vi "Modem Status data gathering Loop.vi"(1 "Loop ID":T1=enum."Var Handling-From PCP", 11 "error in":errorcluster) -> ()   [LabVIEW 2011]
uses:
  Application Structure/Loop ID.ctl
  Tool/Variable List Tool Analog.ctl
  Tool/Variable List Tool Digital.ctl
  Common/Variable List Common Digital.ctl
  Common/Variable List Common Analog.ctl
  Action Analog Handler.ctl
  Modem Status/Variable List Modem Status Digital.ctl
  Modem Status/Variable List Modem Status Analog.ctl
  Status Digitalish.ctl
  emi Lib/System 01/0 - General/App/Loop control 2/Private/_emi_ SMLoop start condition.vi
  emi Lib/System 01/0 - General/App/Loop control 2/Private/_emi_ SMLoop Error Check.vi
  emi Lib/Basic/0 - General/Error/emi_Is Error.vi
  emi Lib/System 01/0 - General/App/Loop control 2/Private/_emi_SMLoop Register new.vi
  emi Lib/System 01/0 - General/S&E reporting/emi_Send S&E Error message.vi
  emi Lib/Basic/0 - General/Error/emi_ Is Error state.vi
  emi Lib/System 01/0 - General/emi_Read System ID.vi
  emi Lib/System 01/0 - General/App/Loop control/Private/_emi_GFV Loop Linking.vi
  emi Lib/System 01/0 - General/App/Loop control/Private/_emi_GFV Loop Enable.vi
  emi Lib/System 01/0 - General/App/Loop control 2/Private/_emi_ SMLoop Restart.vi
  emi Lib/System 01/0 - General/App/Private/_emi_GFV App Close.vi
  emi Lib/System 01/0 - General/App/Loop control 2/Private/_emi_ SMLoop Restart Counter.vi
  emi Lib/System 01/0 - General/App/Loop control/Private/_emi_GFV Loop Running.vi
  emi Lib/System 01/0 - General/Private/_emi_GFV System ID.vi
  emi Lib/System 01/0 - General/S&E reporting/Private/_emi_S&E Q Generator.vi
  <vilib>/Utility/error.llb/Clear Errors.vi
  emi Lib/System 01/0 - General/App/Loop control/Private/_emi_GFV stop a loop so it can reset.vi
  <vilib>/Utility/VariantDataType/GetNumericInfo.vi
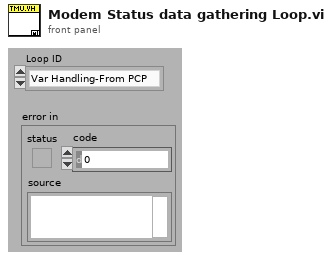
[diagram p1: front panel]
types:
  T1 = typedef "Loop ID.ctl" = enum16{"Main-QSM", "Main-Dialog", "Main-Ind Upd", "Main-Graph Upd", "Main-Debug", "Main-DebugW1", "Main-DebugW2", "Main-SE Handler", "Interface-PCP", "Interface-CANbus", "Interface-Modem", "Var Handling-Beat", "Var Handling-From PCP", "Var Handling-File storage", "Var Handling-From Simulator", "GUI-GrphW Mast", "GUI-GrphW Slav", "SIM-Tool W1", "SIM-Tool W2", "Alm-Sound", "LEIN-motor", "Tool data gatherer Qer", "Tool Data LEIN STAT2 dekoder", "Indicator Value Update", "Tool STAT2 dedicated reader", "Tool ID handler", "Detail View L1", "Detail View L2", "Main display enable view", "Sequence runner", "Voltage setpoint", "Resistance setpoint", "Stroker Wizard L1", "Stroker Wizard L2", "Alarm Handling", "Annotations Tip Strip", "Magna Interface", "Modem Status", "Var Handling - Modem Status", "Power interface detector"}
  T2 = typedef "Variable List Tool Analog.ctl" = enum16{"Tool Max Temperature", "Tool (Controller) Temperature", "Tool Supply Voltage", "Tool (Controller) Current", "Tool Acceleration X", "Tool Acceleration Y", "Tool Acceleration Z", "Tool Acceleration Sum", "Tool Inclination", "Tool Rotation", "Tool GP Sensor 1", "Tool GP Sensor 2", "Tool (Pressure 1) Temperature", "Tool Pressure 1 RAW", "Tool (Pressure 2) Temperature", "Tool Pressure 2 RAW", "Tool (Solenoid) Temperature", "Tool Solenoid Position", "PSU Temp", "Head Voltage", "PSU Main Voltage out", "PSU Main Current out", "Upper Tension Sub Temp", "Tool Upper Tension Sub Raw", "Lower Tension Sub Temp", "Tool Lower Tension Sub Raw", "Tool Var27 - Reserved", "Tool Var28 - Reserved", "Tool Var29 - Reserved", "Tool Var30 - Reserved", "Stroke Extension", "Stroke In Force", "Stroke Out Force", "Stroke Force", "Stroker Pressure 1", "Stroker Pressure 2", "Stroker Upper Tension Sub", "Stroker Lower Tension Sub", "Stroker Var09 - Reserved", "Stroker Var10 - Reserved", "Tractor Upper Tension Sub", "Tractor Lower Tension Sub", "Tractor Var03 - Reserved", "Tractor Var04 - Reserved", "Tool Temperature sensor", "Tool Motor Voltage", "Tool Motor Current", "Tool Motor Torque", "Tool weight on bit", "Tool Motor RPM"}
  T3 = typedef "Variable List Tool Digital.ctl" = enum16{"Tool Error Controller", "Tool Stopped Controller", "Tool Relay 1", "Tool Relay 2", "Tool Both Relays", "Tool node Pressure 1", "Tool Error Pressure 1", "Tool Stopped Pressure 1", "Tool node Pressure 2", "Tool Error Pressure 2", "Tool Stopped Pressure 2", "Tool node Solenoid", "Tool Error Solenoid", "Tool Stopped Solenoid", "Tool Solenoid 1", "Tool Solenoid 2", "Tool Solenoid 3", "Tool node PSU", "Tool Error PSU", "Tool Stopped PSU", "Upper Tension Sub", "Tool Error Upper Tension Sub", "Tool Stopped Upper Tension Sub", "Lower Tension Sub", "Tool Error Lower Tension Sub", "Tool Stopped Lower Tension Sub", "Stroke Target seeking", "Stroke Moving Out", "Stroke Moving Inn", "Stroke valves set for Out", "Stroke valves set for In", "Stroke In (force)", "Stroke Out (force)", "Stroke Force decreasing(in)", "Stroke Force decreasing(out)", "Stroke Force change not correct", "Stroke SLIPS established P1", "Stroke SLIPS established P2", "Stroke SLIPS established", "Stroke Pressure Monitor Ongoing", "Stroke Pressure Monitor Ending ", "Tool Stroke enable Valve", "Tool Stroke direction Valve", "Tool Anchor Valve", "Stroker Var19 - Reserved", "Stroker Var20 - Reserved", "Stroker Var21 - Reserved", "Stroker Var22 - Reserved", "Stroker Var23 - Reserved", "Stroker Var24 - Reserved", "Tractor Var1 - Reserved", "Tractor Var2 - Reserved", "Tractor Var3 - Reserved", "Tractor Var4 - Reserved", "Tractor Var5 - Reserved", "Tractor Var6 - Reserved", "Tractor Var7 - Reserved", "Tractor Var8 - Reserved", "Oil filling mode", "Mill Bit Direction", "Position control", "Anchor", "Driller Var5 - Reserved", "Driller Var6 - Reserved", "Driller Var7 - Reserved", "Driller Var8 - Reserved"}
  T4 = typedef "Variable List Common Digital.ctl" = enum16{"PCP Connected", "PCP PC Control", "HV PSU connected", "HV PSU HV Active", "Modem Connected", "Tool Connected", "CanBus interface"}
  T5 = typedef "Variable List Common Analog.ctl" = enum16{"HVPSU Head Voltage", "HVPSU TS Voltage", "HVPSU Current", "PCP Cable Resistance", "Winch Depth", "Winch Line Speed", "Winch Wire Tension"}
  T6 = typedef "Action Analog Handler.ctl" = enum16{"GET value", "GET Single Frequenzy", "GET All Values", "GET Waveform", "Get Numb Var", "SET Value", "START Buffer", "REG Variable", "BUF size(total antal sekund)", "PULS", "Get a Value at time", "Set initial waveform"}
  T7 = typedef "Status Digitalish.ctl" = enum16{"NA", "False", "True"}
  T8 = typedef "_emi_ SMLoop sates.ctl" = enum16{"Init", "Standby", "Start", "Normal Operation", "Stop", "Error Handling", "End", "Post"}
  T9 = cluster{"notifier out":refnum<notifier>, "Ana com":i32, "Dig com":i32}
  T10 = typedef "Options  All pages and custom.ctl" = cluster{"P 1 (App)":T11, "P 2":T12, "P 3":T13, "P 4":T16, "P 5":T21, "P 6 (Err)":T22, "P 7 (Expert)":T23, "P 8 (Depth)":T25, "C 1":T26, "C 2":T27}
  T11 = typedef "Options Page 1 (App).ctl" = cluster{"Result files":path, "PCP Interface":string, "Tractor/Stroker Interface":string, "Tractor Interface":string, "Modem Status Interface":string, "Audible Alarm":bool, "Force alarm on Technical":bool, "Force alarm on HH":bool, "Force alarm on LL":bool, "Force alarm on H":bool, "Force alarm on L":bool}
  T12 = typedef "Options Page 2.ctl" = cluster{"Solenoid & Relay latching time":u16, "Tractor relay 1":dbl, "Tractor relay 2":dbl, "Tractor Solenoid limit":dbl}
  T13 = typedef "Options Page 3.ctl" = cluster{"Min resistance":dbl, "Max resistance":dbl, "Head voltage range":T14, "Max voltage jump":dbl, "Maximum resistance change":dbl, "Start Telemetry Voltage":dbl, "Start Telemetry Timeout":dbl, "Start Motor Voltage":dbl, "Stop Motor Voltage":dbl, "Pass Mode Warning Voltage":dbl, "Relay Switch Voltage":dbl, "Relay Status Loss Voltage":dbl, "Samples to average":i32, "PSU type DO NOT USE":T15, "Magna OVP":dbl, "Magna Current Limit":dbl}
  T14 = typedef "PCP type List.ctl" = enum16{"0 - 350V", "0 - 450V", "0 - 600V"}
  T15 = typedef "PSU Type.ctl" = enum16{"Unipower", "Magna 8.3A", "Magna 12A", "None"}
  T16 = typedef "Options Page 4.ctl" = cluster{"Solenoid & Relay latching time":u16, "Stroker relay 1":dbl, "Stroker Relay 2":dbl, "Stroker Solenoid limit":dbl, "Force det.":T17, "Stroke force lim.":dbl, "Anchor Enabled Pressure":dbl, "Tacometer puls":dbl, "Default anchor behavior":T18, "Default stroker behavior":T19, "Default stroker force limit (tonne)":dbl, "Slips Size":T20}
  T17 = typedef "Stroke force selector.ctl" = enum16{"Stroke in = node 1", "Strok out = node 1"}
  T18 = typedef "Default anchor behavior.ctl" = enum16{"Do nothing", "Set Anchor", "Release Anchor"}
  T19 = typedef "Default stroker behavior.ctl" = enum16{"Do nothing", "Stop", "Go Out", "Go In"}
  T20 = typedef "Slips Type Radio.ctl" = enum32{"No Selection", "338 MRS", "3,9 MRS"}
  T21 = typedef "Options Page 5.ctl" = cluster{"Solenoid & Relay latching time":u16, "Driller relay 1":dbl, "Driller Relay 2":dbl, "Driller  Solenoid limit":dbl}
  T22 = typedef "Options Page 6 (Err).ctl" = cluster{"Error and event files":path}
  T23 = typedef "Options Page 7 (Expert).ctl" = cluster{"Show Debug":bool, "Log debug messages":bool, "Additional debug messages":bool, "Start Beagle with Simulator data":bool, "Workshop mode":bool, "Modem baud":u16, "enumCANCOM":bool, "Modem sim":T24, "Telemetry Timeout Disable":i32, "Buffer size":i32, "Upd regular data":bool, "Cable comp":cluster{"VMOD1 Voltage(V)":dbl, "VMOD2 Voltage(V)":dbl}}
  T24 = typedef "Modem simulation setup.ctl" = cluster{"Modem dealay sim":bool, "Sim baud Tx":u16, "Bit Error fraction Tx":dbl, "Sim baud Rx":u16, "Bit Error fraction Rx":dbl}
  T25 = typedef "Options Page 8 (Depth).ctl" = cluster{"Winch Spool Circumference":dbl, "Winch Pulses per Revolution":dbl, "Current Depth":dbl}
  T26 = typedef "Options Custom 1.ctl" = cluster{"Depth Updated":bool, "Depth Offset":dbl}
  T27 = typedef "Options Custom 2.ctl" = cluster{"Placeholder":bool}
  T28 = typedef "Fixed Analog Channel Definition.ctl" = cluster{"ID":u16, "Name":string, "Quantity":T29, "Unit":string, "Maximum upd":T30, "Comment":string, "Help file Name":string, "Help file Section ":string, "Category":T31, "User adjustable Scaling":bool, "Default Scaling":T32, "Default Unit":i32, "Classification":T33}
  T29 = typedef "Quantity enum.ctl" = enum16{"NA", "Acceleration", "Angle", "Current", "Force", "Distance", "Pressure", "Resistance", "Rotational Speed", "Speed", "Temperature", "Tension", "Torque", "Voltage", "Weight"}
  T30 = typedef "Update frequensies.ctl" = enum16{"2 Hz", "1 Hz", "0.1 Hz"}
  T31 = typedef "Channel catagory Enum.ctl" = enum16{"No Category", "Power", "Temperature", "Pressure"}
  T32 = typedef "Scaling.ctl" = cluster{"Gain":dbl, "Offset":dbl}
  T33 = typedef "Channel Classification Enum.ctl" = enum16{"Basic", "Advanced", "Expert", "Unused"}
  T34 = typedef "Fixed Digital Channel Definition.ctl" = cluster{"ID":u16, "Name":string, "NA Text":string, "Off Text":string, "On Text":string, "Maximum upd":T30, "Comment":string, "Help file Name":string, "Help file Section ":string, "Catagory":T31, "In use":bool}
  T35 = typedef "Variable List Modem Status Digital.ctl" = enum16{"TMU_LINK_STATUS"}
  T36 = typedef "Variable List Modem Status Analog.ctl" = enum16{"TS_Signal_Quality", "TS_PCB_Temp", "TS_Gain", "DH_Signal_Quality", "DH_PCB_Temp", "DH_Gain", "Link_Status"}
  T37 = typedef "Modem Status Raw Analog Data Cluster.ctl" = cluster{"PCB Temp TS":dbl, "PCB Temp DH":dbl, "RX Gain TS":dbl, "RX Gain DH":dbl, "Signal Quality TS":dbl, "Signal Quality DH":dbl, "Numeric Link Status":dbl, "Link Status":bool}
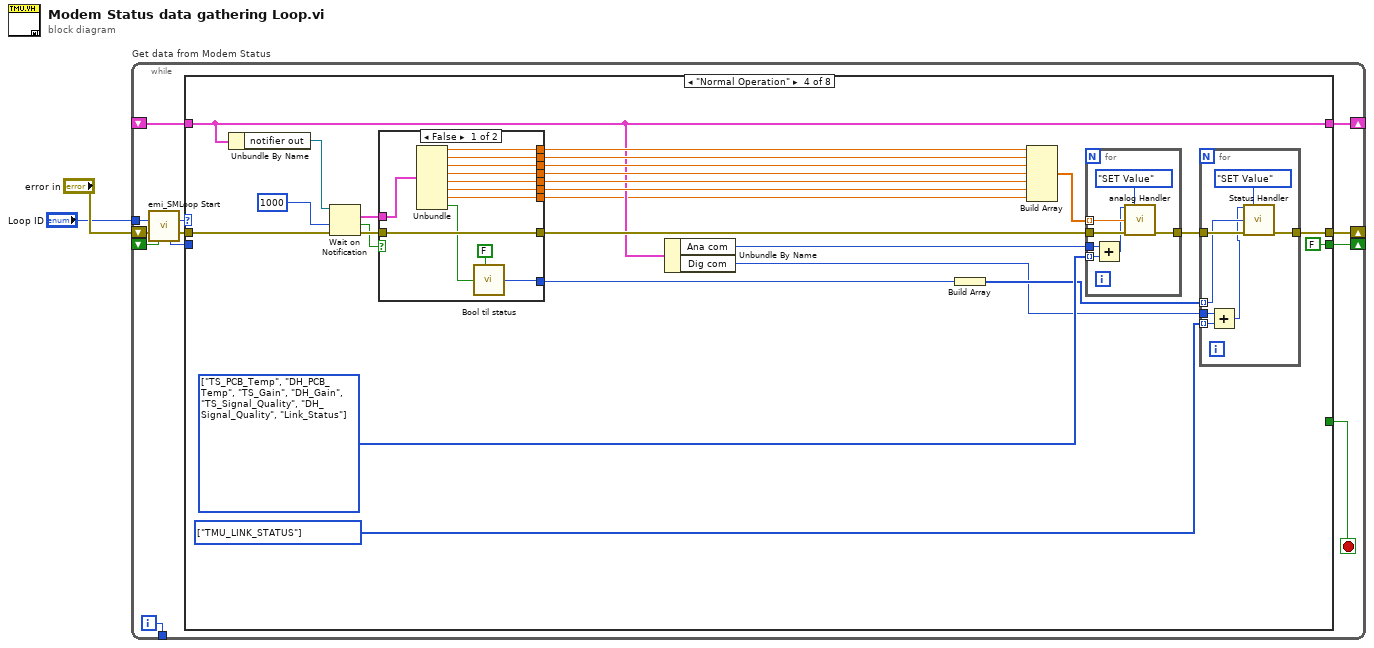
[diagram p0: block diagram]
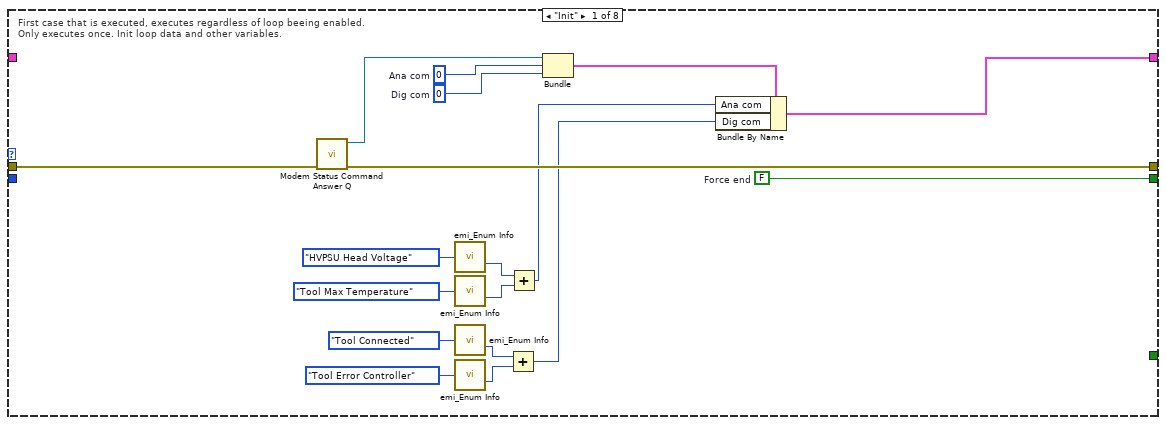
[diagram p2: hidden frame]
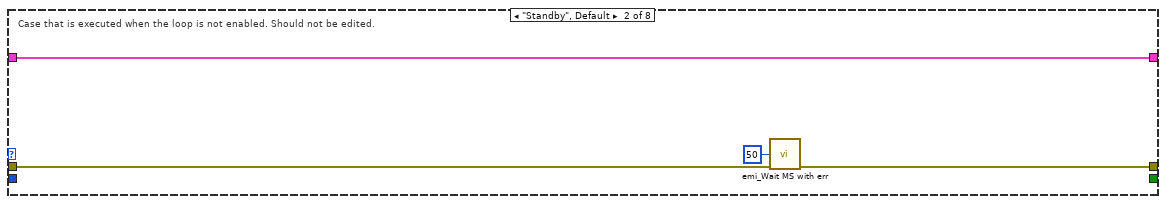
[diagram p3: hidden frame]
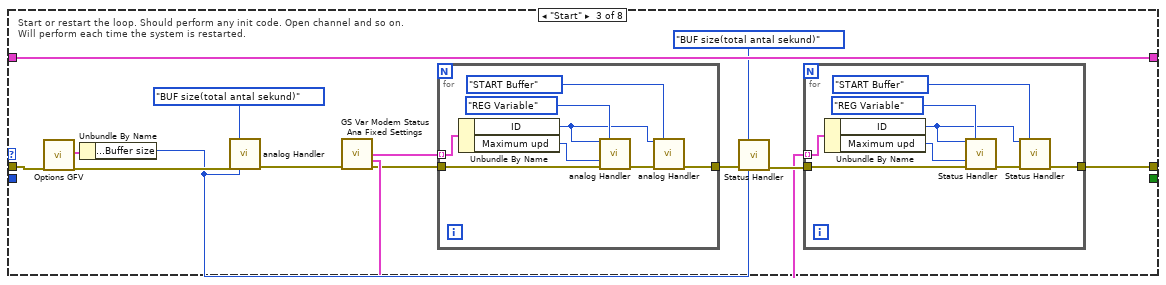
[diagram p4: hidden frame]
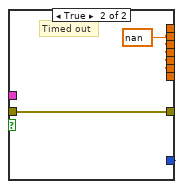
[diagram p5: hidden frame]
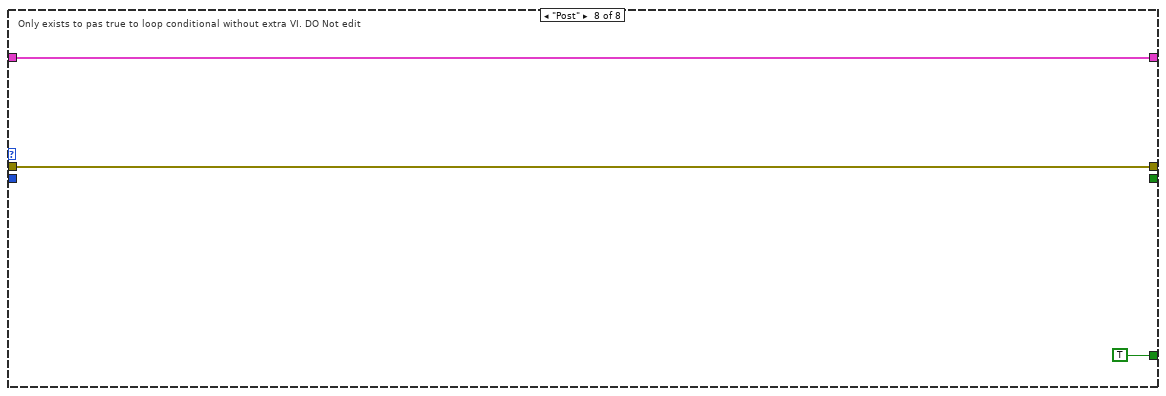
[diagram p9: hidden frame]
diagram:
  n1 = while "Get data from Modem Status" {
    shift-right: [w14] -> _
    shift-left: _ -> [w11]
    tunnel: [w12] -> _
    shift-right: [w10] -> _
    shift-left: _ -> [w5]
    tunnel: "Loop ID" -> [w6]
    shift-right: [w3] -> _
    shift-left: "error in" -> [w9]
    i -> [w12]
    stop <- w13 stop-if-true
    n2 = call "emi_SMLoop Start.vi"("Loop ID"=w6, "error in (no error)"=w9, "Force Stop(F)"=w5) -> ("Loop command"=w7:T8, "error out"=w8:errorcluster, "Loop ID out"=w4:i32)  [unwired: 10 in]
    n3 = case shown="\"Normal Operation\"" w7 {
      tunnel: [w19 w33 w50 w70 w121 w124 w125 w128] -> w14
      tunnel: [_ _ _ _ _ _ _ TRUE] -> w13
      tunnel: w8 -> [w31 w35 w48 w91 w122 w123 w126 w129]
      tunnel: [w30 w34 w41 w89 w122 w123 w126 w129] -> w3
      tunnel: w11 -> [_ w33 w50 w70 w121 w124 w125 w128]
      tunnel: [w32 _ _ FALSE ("Force End") _ _ _ _] -> w10
      tunnel: w4 -> [_ _ _ _ _ _ _ _]
      frame "Init" {
        w27 = 0  # Dig com
        w28 = 0  # Ana com
        w32 = FALSE  # Force end
        # "First case that is executed, executes regardless of loop beeing enabled.\nOnly executes once. Init loop data and other variables."
        n4 = call "Modem Status Command Answer Q.vi"("error in (no error)"=w31) -> ("error out"=w30:errorcluster, "notifier out"=w29:refnum<notifier>)  [unwired: 9 in]
        n5 = call "emi_Enum Info.vi"("Enum"=Variable_List_Common_Analog."HVPSU Head Voltage" ("Action")) -> ("Numb Elements"=w24:i32)  [unwired: 11 in, 3 out]
        n6 = call "emi_Enum Info.vi"("Enum"=Variable_List_Tool_Analog."Tool Max Temperature") -> ("Numb Elements"=w23:i32)  [unwired: 11 in, 3 out]
        n7 = call "emi_Enum Info.vi"("Enum"=Variable_List_Common_Digital."Tool Connected" ("Action")) -> ("Numb Elements"=w22:i32)  [unwired: 11 in, 3 out]
        n8 = call "emi_Enum Info.vi"("Enum"=Variable_List_Tool_Digital."Tool Error Controller" ("Variable")) -> ("Numb Elements"=w21:i32)  [unwired: 11 in, 3 out]
        n9 = Add(x=w22, y=w21) -> (x+y=w17:i32)
        n10 = Add(x=w24, y=w23) -> (x+y=w18:i32)
        n11 = Bundle("notifier out"=w29, "Ana com"=w28, "Dig com"=w27) -> (w20:T9)  [unwired: 1 in]
        n12 = Bundle By Name(cluster=w20, "Ana com"=w18, "Dig com"=w17) -> (w19:T9)
      }
      frame "Standby", Default {
        # "Case that is executed when the loop is not enabled. Should not be edited."
        n13 = call "emi_Wait MS with err.vi"("milliseconds to wait(0)"=u32 50, "error in (no error)"=w35) -> ("error out"=w34:errorcluster)  [unwired: 13 in]
      }
      frame "Start" {
        # "Start or restart the loop. Should perform any init code. Open channel and so on. \nWill perform each time the system is restarted."
        n14 = call "Options GFV.vi"("error in (no error)"=w48) -> ("Options"=w46:T10, "error out"=w47:errorcluster)  [unwired: 16 in, 1 out]
        n15 = Unbundle By Name(w46) -> ("P 7 (Expert).Buffer size"=w44:i32)
        n16 = call "analog Handler.vi"("Action"=Action_Analog_Handler."BUF size(total antal sekund)" ("Action(GET)"), "error in (no error)"=w47, "Start tid / buf size"=w44) -> ("error out"=w40:errorcluster)  [unwired: 7 in, 5 out]
        n17 = call "GS Var Modem Status Ana Fixed Settings.vi"("error in (no error)"=w40) -> ("Modem Status Analog var Fixed out"=w39:T28[], "Modem Status Digital Var Fixed out"=w38:T34[], "error out"=w37:errorcluster)  [unwired: 12 in]
        n18 = for {
          tunnel: [w61] -> w45
          tunnel: w37 -> [w66]
          tunnel: w39 -> [w65] mode=indexing
          n19 = Unbundle By Name(w65) -> ("ID"=w60:u16, "Maximum upd"=w64:T30)
          n20 = call "analog Handler.vi"("Variable Index"=w60, "Action"=Action_Analog_Handler."REG Variable" ("Action(GET)"), "Upd freq"=w64, "error in (no error)"=w66) -> ("error out"=w62:errorcluster)  [unwired: 6 in, 5 out]
          n21 = call "analog Handler.vi"("Variable Index"=w60, "Action"=Action_Analog_Handler."START Buffer" ("Action(GET)"), "error in (no error)"=w62) -> ("error out"=w61:errorcluster)  [unwired: 7 in, 5 out]
        }
        n22 = call "Status Handler.vi"("Action"=Action_Analog_Handler."BUF size(total antal sekund)", "error in (no error)"=w45, "Start tid(buff size"=w44) -> ("error out"=w42:errorcluster)  [unwired: 8 in, 4 out]
        n23 = for {
          tunnel: [w53] -> w41
          tunnel: w42 -> [w58]
          tunnel: w38 -> [w57] mode=indexing
          n24 = Unbundle By Name(w57) -> ("ID"=w52:u16, "Maximum upd"=w56:T30)
          n25 = call "Status Handler.vi"("Variable Index"=w52, "Action"=Action_Analog_Handler."REG Variable" ("Action(GET)"), "Upd freq"=w56, "error in (no error)"=w58) -> ("error out"=w54:errorcluster)  [unwired: 7 in, 4 out]
          n26 = call "Status Handler.vi"("Variable Index"=w52, "Action"=Action_Analog_Handler."START Buffer" ("Action(GET)"), "error in (no error)"=w54) -> ("error out"=w53:errorcluster)  [unwired: 8 in, 4 out]
        }
      }
      frame "Normal Operation" {
        w80 = T35[] [enum."TMU_LINK_STATUS"] items=["TMU_LINK_STATUS"]
        w82 = T36[] [enum."TS_PCB_Temp", enum."DH_PCB_Temp", enum."TS_Gain", enum."DH_Gain", enum."TS_Signal_Quality", enum."DH_Signal_Quality", enum."Link_Status"] items=["TS_Signal_Quality", "TS_PCB_Temp", "TS_Gain", "DH_Signal_Quality", "DH_PCB_Temp", "DH_Gain", "Link_Status"]
        n27 = Unbundle By Name(w70) -> ("notifier out"=w87:refnum<notifier>)
        n28 = Wait on Notification(notifier=w87, timeout in ms (-1)=1000, error in (no error)=w91) -> (notification=w86:T37, timed out?=w84:bool, error out=w85:errorcluster)  [unwired: 1 in, 1 out]
        n29 = case shown="False" w84 {
          tunnel: w86 -> [w117 _]
          tunnel: w85 -> [w109 w120]
          tunnel: [w114 w118] -> w76
          tunnel: [w113 w118] -> w75
          tunnel: [w112 w118] -> w74
          tunnel: [w116 Status_Digitalish."NA" ("Status")] -> w79
          tunnel: [w115 w118] -> w77
          tunnel: [w111 w118] -> w73
          tunnel: [w110 w118] -> w72
          tunnel: [w109 w120] -> w71
          tunnel: [w106 w118] -> w67
          frame False {
            n30 = Unbundle(w117) -> ("PCB Temp TS"=w115:dbl, "PCB Temp DH"=w114:dbl, "RX Gain TS"=w113:dbl, "RX Gain DH"=w112:dbl, "Signal Quality TS"=w111:dbl, "Signal Quality DH"=w110:dbl, "Numeric Link Status"=w106:dbl, "Link Status"=w107:bool)
            n31 = call "Bool til status.vi"("Force NA(F)"=FALSE, "Boolean"=w107) -> ("Status"=w116:T7)  [unwired: 7 in]
          }
          frame True {
            w118 = nan ("Common TS.V")
            # "Timed out"
          }
        }
        n32 = Unbundle By Name(w70) -> ("Ana com"=w69:i32, "Dig com"=w68:i32)
        n33 = Build Array(w79) -> (w78:T7[])
        n34 = Build Array(w77, w76, w75, w74, w73, w72, w67) -> (w83:dbl[])
        n35 = for {
          tunnel: w71 -> [w105]
          tunnel: [w104] -> w81
          tunnel: w82 -> [w101] mode=indexing
          tunnel: w83 -> [w102] mode=indexing
          tunnel: w69 -> [w100]
          n36 = Add(x=w100, y=w101) -> (x+y=w99:i32)
          n37 = call "analog Handler.vi"("Variable Index"=w99, "Action"=Action_Analog_Handler."SET Value" ("Action(GET)"), "Value"=w102, "error in (no error)"=w105) -> ("error out"=w104:errorcluster)  [unwired: 6 in, 5 out]
        }
        n38 = for {
          tunnel: w81 -> [w98]
          tunnel: [w97] -> w89
          tunnel: w80 -> [w93] mode=indexing
          tunnel: w78 -> [w95] mode=indexing
          tunnel: w68 -> [w94]
          n39 = Add(x=w94, y=w93) -> (x+y=w92:i32)
          n40 = call "Status Handler.vi"("Variable Index"=w92, "Action"=Action_Analog_Handler."SET Value" ("Action(GET)"), "Value"=w95, "error in (no error)"=w98) -> ("error out"=w97:errorcluster)  [unwired: 7 in, 4 out]
        }
      }
      frame "Stop" {
        # "Stop the loop. May be restarted later. Close interfaces and the like"
      }
      frame "Error Handling" {
        # "Loop automaticaly returns here after error is found. If error is cleared, Loop wil continue\nas normal(if was operative when error."
      }
      frame "End" {
        # "Only executes at application end has. Should performa any action the loop needs to finnish. \nExecutes only once."
      }
      frame "Post" {
        # "Only exists to pas true to loop conditional without extra VI. DO Not edit"
      }
    }
  }
